vi "core_is_specific_controll.vi"(7 "specific class":T1, 10 "ctrl ref":refnum<vi>) -> (2 "is specific control?":bool)   [LabVIEW 2015]
uses:
  core_controls_children_names.ctl
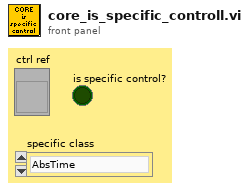
[diagram p1: front panel]
types:
  T1 = typedef "core_controls_children_names.ctl" = enum16{"AbsTime", "ActiveXContainer", "Array", "Boolean", "Cluster", "RadioButtonsControl", "ColorBox", "DigitalTable", "GraphChart", "IntensityChart", "IntensityGraph", "MixedSignalGraph", "WaveformChart", "WaveformGraph", "DigitalGraph", "XYGraph", "IOName", "DAQChannelName", "DAQmxName", "IVILogicalName", "VISAResourceName", "LabVIEWClassControl", "ListBox", "LVVariant", "MixedCheckbox", "MulticolumnListbox", "MultiSegmentPipe", "Numeric", "ColorRamp", "Digital", "NamedNumeric", "Enum", "Ring", "NumericWithScale", "Knob", "Slide", "PageSelector", "TabControl", "Path", "Picture", "Pixmap", "RefNum", "LVObjectRefNum", "VIRefNum", "TypedRefNum", "DataValRefNum", "SceneGraphDisplay", "Scrollbar", "String", "ComboBox", "SubPanel", "Table", "TreeControl", "WaveformData"}
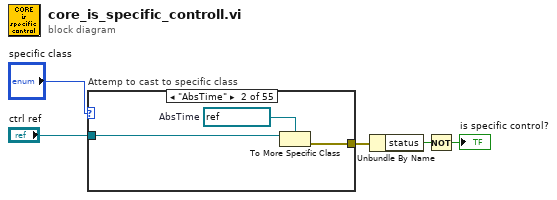
[diagram p0: block diagram]
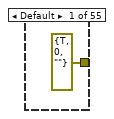
[diagram p2: hidden frame]
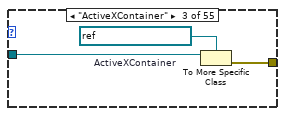
[diagram p3: hidden frame]
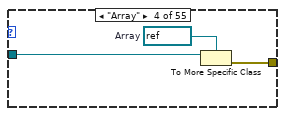
[diagram p4: hidden frame]
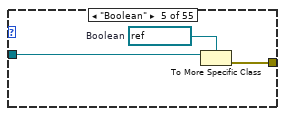
[diagram p5: hidden frame]
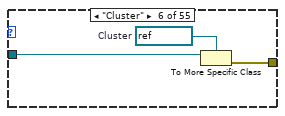
[diagram p6: hidden frame]
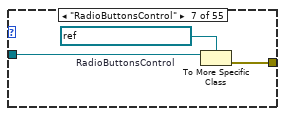
[diagram p7: hidden frame]
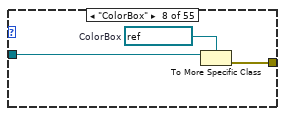
[diagram p8: hidden frame]
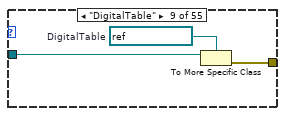
[diagram p9: hidden frame]
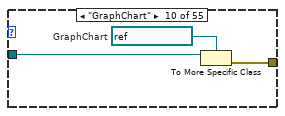
[diagram p10: hidden frame]
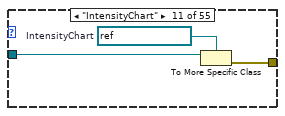
[diagram p11: hidden frame]
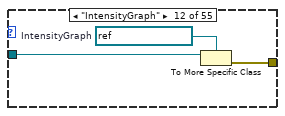
[diagram p12: hidden frame]
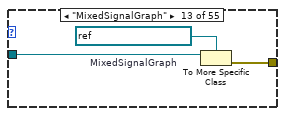
[diagram p13: hidden frame]
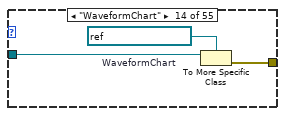
[diagram p14: hidden frame]
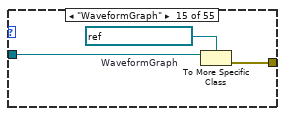
[diagram p15: hidden frame]
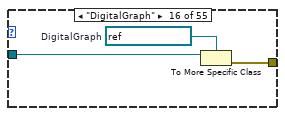
[diagram p16: hidden frame]
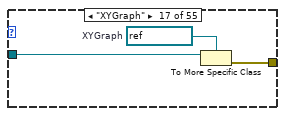
[diagram p17: hidden frame]
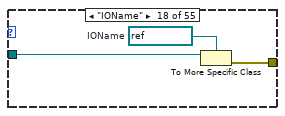
[diagram p18: hidden frame]
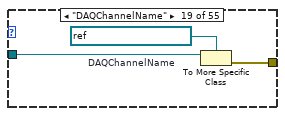
[diagram p19: hidden frame]
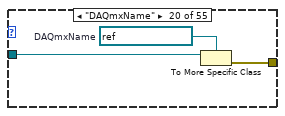
[diagram p20: hidden frame]
diagram:
  n1 = case "Attemp to cast to specific class" shown="\"AbsTime\"" "specific class" {
    tunnel: "ctrl ref" -> [_ w9 w12 w14 w17 w20 w24 w26 w29 w32 w35 w38 w41 w45 w48 w51 w54 w57 w60 w63 w66 w69 w72 w75 w78 w81 w84 w87 w90 w93 w96 w99 w102 w105 w108 w111 w114 w117 w120 w123 w126 w129 w132 w135 w138 w141 w144 w147 w150 w153 w156 w159 w162 w165 w168]
    tunnel: [errorcluster {"status"=TRUE, "code"=0, "source"=""} ("error constant") w7 w10 w13 w16 w19 w22 w25 w28 w31 w34 w37 w40 w44 w47 w50 w53 w56 w59 w62 w65 w68 w71 w74 w77 w80 w83 w86 w89 w92 w95 w98 w101 w104 w107 w110 w113 w116 w119 w122 w125 w128 w131 w134 w137 w140 w143 w146 w149 w152 w155 w158 w161 w164 w167] -> w2
    frame Default {
    }
    frame "AbsTime" {
      w8 = refnum<vi> refnum  # AbsTime
      n2 = To More Specific Class(target class=w8, reference=w9) -> (error out=w7:errorcluster)  [unwired: 1 in, 1 out]
    }
    frame "ActiveXContainer" {
      w11 = refnum<vi> refnum  # ActiveXContainer
      n3 = To More Specific Class(target class=w11, reference=w12) -> (error out=w10:errorcluster)  [unwired: 1 in, 1 out]
    }
    frame "Array" {
      w15 = refnum<vi> refnum  # Array
      n4 = To More Specific Class(target class=w15, reference=w14) -> (error out=w13:errorcluster)  [unwired: 1 in, 1 out]
    }
    frame "Boolean" {
      w18 = refnum<vi> refnum  # Boolean
      n5 = To More Specific Class(target class=w18, reference=w17) -> (error out=w16:errorcluster)  [unwired: 1 in, 1 out]
    }
    frame "Cluster" {
      w21 = refnum<vi> refnum  # Cluster
      n6 = To More Specific Class(target class=w21, reference=w20) -> (error out=w19:errorcluster)  [unwired: 1 in, 1 out]
    }
    frame "RadioButtonsControl" {
      w23 = refnum<vi> refnum  # RadioButtonsControl
      n7 = To More Specific Class(target class=w23, reference=w24) -> (error out=w22:errorcluster)  [unwired: 1 in, 1 out]
    }
    frame "ColorBox" {
      w27 = refnum<vi> refnum  # ColorBox
      n8 = To More Specific Class(target class=w27, reference=w26) -> (error out=w25:errorcluster)  [unwired: 1 in, 1 out]
    }
    frame "DigitalTable" {
      w30 = refnum<vi> refnum  # DigitalTable
      n9 = To More Specific Class(target class=w30, reference=w29) -> (error out=w28:errorcluster)  [unwired: 1 in, 1 out]
    }
    frame "GraphChart" {
      w33 = refnum<vi> refnum  # GraphChart
      n10 = To More Specific Class(target class=w33, reference=w32) -> (error out=w31:errorcluster)  [unwired: 1 in, 1 out]
    }
    frame "IntensityChart" {
      w36 = refnum<vi> refnum  # IntensityChart
      n11 = To More Specific Class(target class=w36, reference=w35) -> (error out=w34:errorcluster)  [unwired: 1 in, 1 out]
    }
    frame "IntensityGraph" {
      w39 = refnum<vi> refnum  # IntensityGraph
      n12 = To More Specific Class(target class=w39, reference=w38) -> (error out=w37:errorcluster)  [unwired: 1 in, 1 out]
    }
    frame "MixedSignalGraph" {
      w42 = refnum<vi> refnum  # MixedSignalGraph
      n13 = To More Specific Class(target class=w42, reference=w41) -> (error out=w40:errorcluster)  [unwired: 1 in, 1 out]
    }
    frame "WaveformChart" {
      w43 = refnum<vi> refnum  # WaveformChart
      n14 = To More Specific Class(target class=w43, reference=w45) -> (error out=w44:errorcluster)  [unwired: 1 in, 1 out]
    }
    frame "WaveformGraph" {
      w46 = refnum<vi> refnum  # WaveformGraph
      n15 = To More Specific Class(target class=w46, reference=w48) -> (error out=w47:errorcluster)  [unwired: 1 in, 1 out]
    }
    frame "DigitalGraph" {
      w49 = refnum<vi> refnum  # DigitalGraph
      n16 = To More Specific Class(target class=w49, reference=w51) -> (error out=w50:errorcluster)  [unwired: 1 in, 1 out]
    }
    frame "XYGraph" {
      w52 = refnum<vi> refnum  # XYGraph
      n17 = To More Specific Class(target class=w52, reference=w54) -> (error out=w53:errorcluster)  [unwired: 1 in, 1 out]
    }
    frame "IOName" {
      w55 = refnum<vi> refnum  # IOName
      n18 = To More Specific Class(target class=w55, reference=w57) -> (error out=w56:errorcluster)  [unwired: 1 in, 1 out]
    }
    frame "DAQChannelName" {
      w58 = refnum<vi> refnum  # DAQChannelName
      n19 = To More Specific Class(target class=w58, reference=w60) -> (error out=w59:errorcluster)  [unwired: 1 in, 1 out]
    }
    frame "DAQmxName" {
      w61 = refnum<vi> refnum  # DAQmxName
      n20 = To More Specific Class(target class=w61, reference=w63) -> (error out=w62:errorcluster)  [unwired: 1 in, 1 out]
    }
    frame "IVILogicalName" {
      w64 = refnum<vi> refnum  # IVILogicalName
      n21 = To More Specific Class(target class=w64, reference=w66) -> (error out=w65:errorcluster)  [unwired: 1 in, 1 out]
    }
    frame "VISAResourceName" {
      w67 = refnum<vi> refnum  # VISAResourceName
      n22 = To More Specific Class(target class=w67, reference=w69) -> (error out=w68:errorcluster)  [unwired: 1 in, 1 out]
    }
    frame "LabVIEWClassControl" {
      w70 = refnum<vi> refnum  # LabVIEWClassControl
      n23 = To More Specific Class(target class=w70, reference=w72) -> (error out=w71:errorcluster)  [unwired: 1 in, 1 out]
    }
    frame "ListBox" {
      w73 = refnum<vi> refnum  # ListBox
      n24 = To More Specific Class(target class=w73, reference=w75) -> (error out=w74:errorcluster)  [unwired: 1 in, 1 out]
    }
    frame "LVVariant" {
      w76 = refnum<vi> refnum  # LVVariant
      n25 = To More Specific Class(target class=w76, reference=w78) -> (error out=w77:errorcluster)  [unwired: 1 in, 1 out]
    }
    frame "MixedCheckbox" {
      w79 = refnum<vi> refnum  # MixedCheckbox
      n26 = To More Specific Class(target class=w79, reference=w81) -> (error out=w80:errorcluster)  [unwired: 1 in, 1 out]
    }
    frame "MulticolumnListbox" {
      w82 = refnum<vi> refnum  # MulticolumnListbox
      n27 = To More Specific Class(target class=w82, reference=w84) -> (error out=w83:errorcluster)  [unwired: 1 in, 1 out]
    }
    frame "MultiSegmentPipe" {
      w85 = refnum<vi> refnum  # MultiSegmentPipe
      n28 = To More Specific Class(target class=w85, reference=w87) -> (error out=w86:errorcluster)  [unwired: 1 in, 1 out]
    }
    frame "Numeric" {
      w88 = refnum<vi> refnum  # Numeric
      n29 = To More Specific Class(target class=w88, reference=w90) -> (error out=w89:errorcluster)  [unwired: 1 in, 1 out]
    }
    frame "ColorRamp" {
      w91 = refnum<vi> refnum  # ColorRamp
      n30 = To More Specific Class(target class=w91, reference=w93) -> (error out=w92:errorcluster)  [unwired: 1 in, 1 out]
    }
    frame "Digital" {
      w94 = refnum<vi> refnum  # Digital
      n31 = To More Specific Class(target class=w94, reference=w96) -> (error out=w95:errorcluster)  [unwired: 1 in, 1 out]
    }
    frame "NamedNumeric" {
      w97 = refnum<vi> refnum  # NamedNumeric
      n32 = To More Specific Class(target class=w97, reference=w99) -> (error out=w98:errorcluster)  [unwired: 1 in, 1 out]
    }
    frame "Enum" {
      w100 = refnum<vi> refnum  # Enum
      n33 = To More Specific Class(target class=w100, reference=w102) -> (error out=w101:errorcluster)  [unwired: 1 in, 1 out]
    }
    frame "Ring" {
      w103 = refnum<vi> refnum  # Ring
      n34 = To More Specific Class(target class=w103, reference=w105) -> (error out=w104:errorcluster)  [unwired: 1 in, 1 out]
    }
    frame "NumericWithScale" {
      w106 = refnum<vi> refnum  # NumericWithScale
      n35 = To More Specific Class(target class=w106, reference=w108) -> (error out=w107:errorcluster)  [unwired: 1 in, 1 out]
    }
    frame "Knob" {
      w109 = refnum<vi> refnum  # Knob
      n36 = To More Specific Class(target class=w109, reference=w111) -> (error out=w110:errorcluster)  [unwired: 1 in, 1 out]
    }
    frame "Slide" {
      w112 = refnum<vi> refnum  # Slide
      n37 = To More Specific Class(target class=w112, reference=w114) -> (error out=w113:errorcluster)  [unwired: 1 in, 1 out]
    }
    frame "PageSelector" {
      w115 = refnum<vi> refnum  # PageSelector
      n38 = To More Specific Class(target class=w115, reference=w117) -> (error out=w116:errorcluster)  [unwired: 1 in, 1 out]
    }
    frame "TabControl" {
      w118 = refnum<vi> refnum  # TabControl
      n39 = To More Specific Class(target class=w118, reference=w120) -> (error out=w119:errorcluster)  [unwired: 1 in, 1 out]
    }
    frame "Path" {
      w121 = refnum<vi> refnum  # Path
      n40 = To More Specific Class(target class=w121, reference=w123) -> (error out=w122:errorcluster)  [unwired: 1 in, 1 out]
    }
    frame "Picture" {
      w124 = refnum<vi> refnum  # Picture
      n41 = To More Specific Class(target class=w124, reference=w126) -> (error out=w125:errorcluster)  [unwired: 1 in, 1 out]
    }
    frame "Pixmap" {
      w127 = refnum<vi> refnum  # Pixmap
      n42 = To More Specific Class(target class=w127, reference=w129) -> (error out=w128:errorcluster)  [unwired: 1 in, 1 out]
    }
    frame "RefNum" {
      w130 = refnum<vi> refnum  # RefNum
      n43 = To More Specific Class(target class=w130, reference=w132) -> (error out=w131:errorcluster)  [unwired: 1 in, 1 out]
    }
    frame "LVObjectRefNum" {
      w133 = refnum<vi> refnum  # LVObjectRefNum
      n44 = To More Specific Class(target class=w133, reference=w135) -> (error out=w134:errorcluster)  [unwired: 1 in, 1 out]
    }
    frame "VIRefNum" {
      w136 = refnum<vi> refnum  # VIRefNum
      n45 = To More Specific Class(target class=w136, reference=w138) -> (error out=w137:errorcluster)  [unwired: 1 in, 1 out]
    }
    frame "TypedRefNum" {
      w139 = refnum<vi> refnum  # TypedRefNum
      n46 = To More Specific Class(target class=w139, reference=w141) -> (error out=w140:errorcluster)  [unwired: 1 in, 1 out]
    }
    frame "DataValRefNum" {
      w142 = refnum<vi> refnum  # DataValRefNum
      n47 = To More Specific Class(target class=w142, reference=w144) -> (error out=w143:errorcluster)  [unwired: 1 in, 1 out]
    }
    frame "SceneGraphDisplay" {
      w145 = refnum<vi> refnum  # SceneGraphDisplay
      n48 = To More Specific Class(target class=w145, reference=w147) -> (error out=w146:errorcluster)  [unwired: 1 in, 1 out]
    }
    frame "Scrollbar" {
      w148 = refnum<vi> refnum  # Scrollbar
      n49 = To More Specific Class(target class=w148, reference=w150) -> (error out=w149:errorcluster)  [unwired: 1 in, 1 out]
    }
    frame "String" {
      w151 = refnum<vi> refnum  # String
      n50 = To More Specific Class(target class=w151, reference=w153) -> (error out=w152:errorcluster)  [unwired: 1 in, 1 out]
    }
    frame "ComboBox" {
      w154 = refnum<vi> refnum  # ComboBox
      n51 = To More Specific Class(target class=w154, reference=w156) -> (error out=w155:errorcluster)  [unwired: 1 in, 1 out]
    }
    frame "SubPanel" {
      w157 = refnum<vi> refnum  # SubPanel
      n52 = To More Specific Class(target class=w157, reference=w159) -> (error out=w158:errorcluster)  [unwired: 1 in, 1 out]
    }
    frame "Table" {
      w160 = refnum<vi> refnum  # Table
      n53 = To More Specific Class(target class=w160, reference=w162) -> (error out=w161:errorcluster)  [unwired: 1 in, 1 out]
    }
    frame "TreeControl" {
      w163 = refnum<vi> refnum  # TreeControl
      n54 = To More Specific Class(target class=w163, reference=w165) -> (error out=w164:errorcluster)  [unwired: 1 in, 1 out]
    }
    frame "WaveformData" {
      w166 = refnum<vi> refnum  # WaveformData
      n55 = To More Specific Class(target class=w166, reference=w168) -> (error out=w167:errorcluster)  [unwired: 1 in, 1 out]
    }
  }
  n56 = Unbundle By Name(w2) -> ("status"=w5:bool)
  n57 = Not(x=w5) -> (.not. x?=→"is specific control?":bool)
